vi "Obtain Request Events.vi"(8 "error in (no error)":errorcluster, 10 "Create New? (F)":bool) -> (0 "error out":errorcluster, 2 "Osciloscope Tektronix Request Events":T1)   [LabVIEW 2020, in "Osciloscope Tektronix.lvlib"]
doc: "This VI Obtains/Creates the Requests events that will be used for other modules to communicate with the module that owns this VI. These Requests events will be accessed only via Public API methods for this module.\n\n<b>NOTE</b>: The contents of this VI are automatically generated and modified by the <b>Tools > Delacor > DQMH</b> utilities. Consider using those utilities instead of making your own modifications to this VI.\n_____\nBased on DQMH Project Template 6.0.0.91."
uses:
  Osciloscope Tektronix.lvlib
  Request Events--cluster.ctl
  Stop Argument--cluster.ctl
  Show Panel Argument--cluster.ctl
  Hide Panel Argument--cluster.ctl
  Show Diagram Argument--cluster.ctl
  Get Module Execution Status Argument--cluster.ctl
  SET COM Port Argument--cluster.ctl
  Initialize Oscilloscope Argument--cluster.ctl
  Close Oscilloscope Argument--cluster.ctl
  AutoSetup Argument--cluster.ctl
  Configure Channel Argument--cluster.ctl
  Reset Argument--cluster.ctl
  Read Waveform Argument--cluster.ctl
  Read Waveform (Reply Payload)--cluster.ctl
  Read Measurement Argument--cluster.ctl
  Read Measurement (Reply Payload)--cluster.ctl
  Read Measurement 2 channels Argument--cluster.ctl
  Read Measurement 2 channels (Reply Payload)--cluster.ctl
panel:
  # "NOTE: The contents of this VI are automatically generated and modified by the Tools > Delacor > DQMH utilities. Consider using those utilities instead of making your own modifications to this VI."
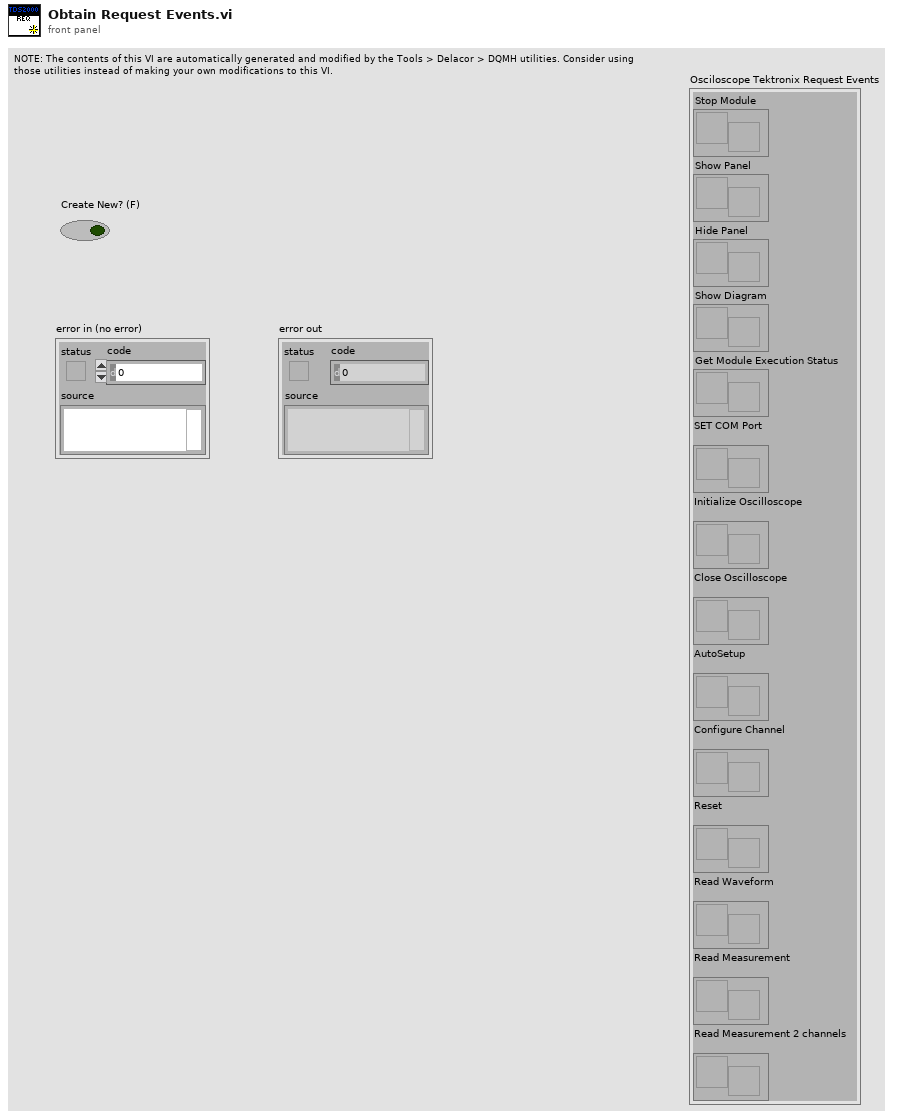
[diagram p1: front panel]
types:
  T1 = typedef "Osciloscope Tektronix.lvlib/Request Events--cluster.ctl" = cluster{"Stop Module":refnum<user-event>, "Show Panel":refnum<user-event>, "Hide Panel":refnum<user-event>, "Show Diagram":refnum<user-event>, "Get Module Execution Status":refnum<user-event>, "SET COM Port":refnum<user-event>, "Initialize Oscilloscope":refnum<user-event>, "Close Oscilloscope":refnum<user-event>, "AutoSetup":refnum<user-event>, "Configure Channel":refnum<user-event>, "Reset":refnum<user-event>, "Read Waveform":refnum<user-event>, "Read Measurement":refnum<user-event>, "Read Measurement 2 channels":refnum<user-event>}
  T2 = typedef "Osciloscope Tektronix.lvlib/Read Measurement 2 channels Argument--cluster.ctl" = cluster{"Module ID":i32, "Wait Notifier":refnum<notifier>, "wait for reply":bool, "Parameters":cluster{"Channel 1 (1: Channel 1)":i32, "Channel 2 (2: Channel 2)":i32, "Measurement Type (0: Phase)":i32}}
  T3 = typedef "Osciloscope Tektronix.lvlib/Read Measurement Argument--cluster.ctl" = cluster{"Module ID":i32, "Wait Notifier":refnum<notifier>, "wait for reply":bool, "Read Parameters":cluster{"Channel (1: Channel 1)":i32, "Measurement Type (0: Frequency)":i32}}
  T4 = typedef "Osciloscope Tektronix.lvlib/Read Waveform Argument--cluster.ctl" = cluster{"Module ID":i32, "Wait Notifier":refnum<notifier>, "wait for reply":bool, "Parameters 3":cluster{"Source (0: Channel 1)":u16, "Timeout (10000 ms)":u32}}
  T5 = typedef "Osciloscope Tektronix.lvlib/Reset Argument--cluster.ctl" = cluster{"Module ID":i32, "Boolean":bool}
  T6 = typedef "Osciloscope Tektronix.lvlib/Configure Channel Argument--cluster.ctl" = cluster{"Module ID":i32, "Boolean":bool, "Parameters":cluster{"Enable Channel (True)":bool, "Channel (0: Channel 1)":i32, "Vertical Coupling (1: DC)":i32, "Probe Attenuation (10: 10X)":i32, "Vertical Range (10.0 V/div)":dbl, "Vertical Offset (0.0 divs)":dbl, "Bandwidth (0: MAX Bandwidth)":i32}}
  T7 = typedef "Osciloscope Tektronix.lvlib/AutoSetup Argument--cluster.ctl" = cluster{"Module ID":i32, "Boolean":bool}
  T8 = typedef "Osciloscope Tektronix.lvlib/Close Oscilloscope Argument--cluster.ctl" = cluster{"Module ID":i32, "Boolean":bool}
  T9 = typedef "Osciloscope Tektronix.lvlib/Initialize Oscilloscope Argument--cluster.ctl" = cluster{"Module ID":i32, "Oscilloscope Type":string}
  T10 = typedef "Osciloscope Tektronix.lvlib/SET COM Port Argument--cluster.ctl" = cluster{"Module ID":i32, "COM":refnum<visa-resource-name>}
  T11 = typedef "Osciloscope Tektronix.lvlib/Get Module Execution Status Argument--cluster.ctl" = cluster{"Module ID":i32, "Running?":bool}
  T12 = typedef "Osciloscope Tektronix.lvlib/Show Diagram Argument--cluster.ctl" = cluster{"Module ID":i32, "Debug?":bool}
  T13 = typedef "Osciloscope Tektronix.lvlib/Show Panel Argument--cluster.ctl" = cluster{"Module ID":i32, "Show Panel?":bool}
  T14 = typedef "Osciloscope Tektronix.lvlib/Hide Panel Argument--cluster.ctl" = cluster{"Module ID":i32, "Hide Panel?":bool}
  T15 = typedef "Osciloscope Tektronix.lvlib/Stop Argument--cluster.ctl" = cluster{"Module ID":i32, "Origin":string, "Exit via Stop Module Req?":bool, "Wait for Module to stop?":bool}
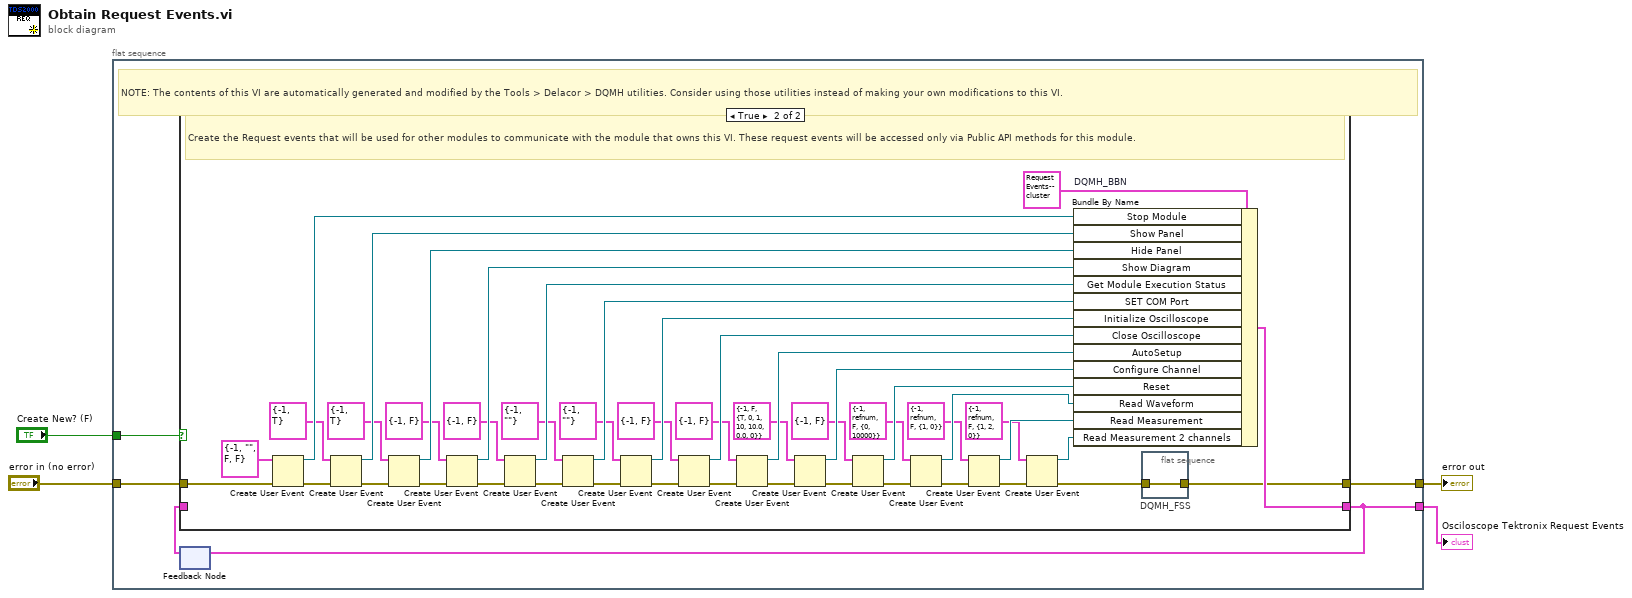
[diagram p0: block diagram]
diagram:
  n1 = flat-sequence {
    tunnel: [w9] -> w4
    tunnel: "error in (no error)" -> [w8]
    tunnel: [w6] -> w2
    tunnel: "Create New? (F)" -> [w5]
    frame #0 {
      # "NOTE: The contents of this VI are automatically generated and modified by the Tools > Delacor > DQMH utilities. Consider using those utilities instead of making your own modifications to this VI."
      n2 = feedback #1() -> (w7:T1)  [unwired: 1 in]
      n3 = case shown="True" w5 {
        tunnel: [w10 w45] -> w9
        tunnel: w8 -> [w10 w57]
        tunnel: [w11 w54] -> w6
        tunnel: w7 -> [w11 _]
        frame False {
        }
        frame True {
          # "Create the Request events that will be used for other modules to communicate with the module that owns this VI. These request events will be accessed only via Public API methods for this module."
          n4 = Create User Event(user event datatype=T15 {"Module ID"=-1, "Origin"="", "Exit via Stop Module Req?"=FALSE, "Wait for Module to stop?"=FALSE} ("Stop Argument"), error in=w57) -> (user event=w55:refnum<user-event>, error out=w52:errorcluster)
          n5 = Create User Event(user event datatype=T13 {"Module ID"=-1, "Show Panel?"=TRUE} ("Show Panel Argument"), error in=w52) -> (user event=w51:refnum<user-event>, error out=w49:errorcluster)
          n6 = Create User Event(user event datatype=T14 {"Module ID"=-1, "Hide Panel?"=TRUE} ("Hide Panel"), error in=w49) -> (user event=w48:refnum<user-event>, error out=w47:errorcluster)
          n7 = Create User Event(user event datatype=T12 {"Module ID"=-1, "Debug?"=FALSE} ("Show Diagram Argument"), error in=w47) -> (user event=w43:refnum<user-event>, error out=w44:errorcluster)
          n8 = Create User Event(user event datatype=T11 {"Module ID"=-1, "Running?"=FALSE} ("Get Module Execution Status Argument"), error in=w44) -> (user event=w40:refnum<user-event>, error out=w41:errorcluster)
          n9 = Create User Event(user event datatype=T10 {"Module ID"=-1, "COM"=""} ("SET COM Port Argument"), error in=w41) -> (user event=w37:refnum<user-event>, error out=w38:errorcluster)
          n10 = Create User Event(user event datatype=T9 {"Module ID"=-1, "Oscilloscope Type"=""} ("Initialize Oscilloscope Argument"), error in=w38) -> (user event=w34:refnum<user-event>, error out=w35:errorcluster)
          n11 = Create User Event(user event datatype=T8 {"Module ID"=-1, "Boolean"=FALSE} ("Close Oscilloscope Argument"), error in=w35) -> (user event=w31:refnum<user-event>, error out=w32:errorcluster)
          n12 = Create User Event(user event datatype=T7 {"Module ID"=-1, "Boolean"=FALSE} ("AutoSetup Argument"), error in=w32) -> (user event=w28:refnum<user-event>, error out=w29:errorcluster)
          n13 = Create User Event(user event datatype=T6 {"Module ID"=-1, "Boolean"=FALSE, "Parameters"={"Enable Channel (True)"=TRUE, "Channel (0: Channel 1)"=0, "Vertical Coupling (1: DC)"=1, "Probe Attenuation (10: 10X)"=10, "Vertical Range (10.0 V/div)"=10.0, "Vertical Offset (0.0 divs)"=0.0, "Bandwidth (0: MAX Bandwidth)"=0}} ("Configure Channel Argument"), error in=w29) -> (user event=w25:refnum<user-event>, error out=w26:errorcluster)
          n14 = Create User Event(user event datatype=T5 {"Module ID"=-1, "Boolean"=FALSE} ("Reset Argument"), error in=w26) -> (user event=w22:refnum<user-event>, error out=w23:errorcluster)
          n15 = Create User Event(user event datatype=T4 {"Module ID"=-1, "Wait Notifier"=refnum, "wait for reply"=FALSE, "Parameters 3"={"Source (0: Channel 1)"=0, "Timeout (10000 ms)"=10000}} ("Read Waveform Argument"), error in=w23) -> (user event=w19:refnum<user-event>, error out=w20:errorcluster)
          n16 = Create User Event(user event datatype=T3 {"Module ID"=-1, "Wait Notifier"=refnum, "wait for reply"=FALSE, "Read Parameters"={"Channel (1: Channel 1)"=1, "Measurement Type (0: Frequency)"=0}} ("Read Measurement Argument"), error in=w20) -> (user event=w16:refnum<user-event>, error out=w17:errorcluster)
          n17 = Create User Event(user event datatype=T2 {"Module ID"=-1, "Wait Notifier"=refnum, "wait for reply"=FALSE, "Parameters"={"Channel 1 (1: Channel 1)"=1, "Channel 2 (2: Channel 2)"=2, "Measurement Type (0: Phase)"=0}} ("Read Measurement 2 channels Argument"), error in=w17) -> (user event=w13:refnum<user-event>, error out=w14:errorcluster)
          n18 = Bundle By Name "DQMH_BBN"(cluster=T1 {"Stop Module"=refnum, "Show Panel"=refnum, "Hide Panel"=refnum, "Show Diagram"=refnum, "Get Module Execution Status"=refnum, "SET COM Port"=refnum, "Initialize Oscilloscope"=refnum, "Close Oscilloscope"=refnum, "AutoSetup"=refnum, "Configure Channel"=refnum, "Reset"=refnum, "Read Waveform"=refnum, "Read Measurement"=refnum, "Read Measurement 2 channels"=refnum} ("output cluster"), "Stop Module"=w55, "Show Panel"=w51, "Hide Panel"=w48, "Show Diagram"=w43, "Get Module Execution Status"=w40, "SET COM Port"=w37, "Initialize Oscilloscope"=w34, "Close Oscilloscope"=w31, "AutoSetup"=w28, "Configure Channel"=w25, "Reset"=w22, "Read Waveform"=w19, "Read Measurement"=w16, "Read Measurement 2 channels"=w13) -> (w54:T1)
          n19 = flat-sequence "DQMH_FSS" {
            tunnel: w14 -> [w58]
            tunnel: [w58] -> w45
            frame #0 {
            }
          }
        }
      }
      n20 = feedback-in #1(w6) -> ()
    }
  }
  "Osciloscope Tektronix Request Events" <- w2
  "error out" <- w4
